vi "Init.vi"(4 "Message Cfg":T2={"EnTermChar"=TRUE, "termChar"=13, "suppEnEnRd"=FALSE, "sendEndEn"=TRUE}, 6 "timeout":u32=1000, 7 "Name":string="CPC", 8 "error in":errorcluster, 9 "serialCfg":T1={"baud rate (9600)"=9600, "data bits (8)"=7, "stop bits (10: 1 bit)"=10, "parity (0:none)"=enum."Even", "flow control (0:none)"=0, "endModeforReads"=2, "endModeforWrites"=2} {"endModeforWrites" items=["None", "Last Bit", "TermChar", "Break"]; "endModeforReads" items=["None", "Last Bit", "TermChar"]; "flow control (0:none)" items=["None", "XON/XOFF", "RTS/CTS", "XON/XOFF & RTS/CTS", "DTR/DSR", "XON/XOFF & DTR/DSR"]; "stop bits (10: 1 bit)" items=["1.0"=10, "1.5"=15, "2.0"=20]; "data bits (8)" min=5 max=8 step=1}, 10 "Port":refnum<visa-resource-name>, 11 "CPC in":refnum<class "CPC.lvclass">) -> (0 "error out":errorcluster, 3 "CPC out":refnum<class "CPC.lvclass">)   [LabVIEW 2014]
uses:
  CPC.lvclass
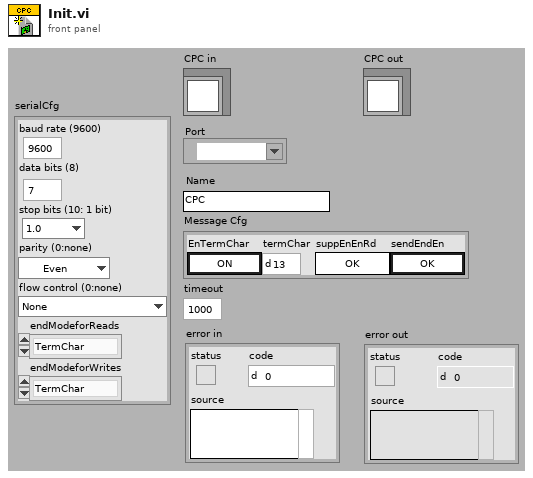
[diagram p1: front panel]
types:
  T1 = cluster{"baud rate (9600)":u32, "data bits (8)":u16, "stop bits (10: 1 bit)":u16, "parity (0:none)":enum16{"None", "Odd", "Even", "Mark", "Space"}, "flow control (0:none)":u16, "endModeforReads":u16, "endModeforWrites":u16}
  T2 = cluster{"EnTermChar":bool, "termChar":u8, "suppEnEnRd":bool, "sendEndEn":bool}
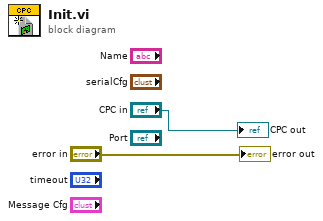
[diagram p0: block diagram]
diagram:
  "error out" <- "error in"
  "CPC out" <- "CPC in"
